vi "KundtsTube.vi"() -> ()   [LabVIEW 2014]
panel:
  out "XY Graph":cluster{"Y":dbl[], "Y":dbl[]}[](graph)=[{"Y"=[10.0, 15.0, 20.0, 25.0, 30.0, 35.0, 40.0, 45.0, 50.0, 55.0, 60.0, 65.0, 70.0, 75.0, 80.0, 85.0, 90.0, 95.0, 100.0, 105.0, 110.0, 115.0, 120.0, 125.0, 130.0, 135.0, 140.0, 145.0, 150.0, 155.0, 160.0, 165.0, 170.0, 175.0, 180.0, 185.0, 190.0, 195.0, 200.0, 205.0, 210.0, 215.0, 220.0, 225.0, 230.0, 235.0, 240.0, 245.0, 250.0, 255.0, 260.0, 265.0, 270.0, 275.0, 280.0, 285.0, 290.0, 295.0, 300.0, 305.0, 310.0, 315.0, 320.0, 325.0, 330.0, 335.0, 340.0, 345.0, 350.0, 355.0, 360.0, 365.0, 370.0, 375.0, 380.0, 385.0, 390.0, 395.0, 400.0, 405.0, 410.0, 415.0, 420.0, 425.0, 430.0, 435.0, 440.0, 445.0, 450.0, 455.0, 460.0, 465.0, 470.0, 475.0, 480.0, 485.0, 490.0, 495.0, 500.0, 505.0, 510.0, 515.0, 520.0], "Y"=[0.04456068816861268, 0.04246761801420257, 0.0029318464951392296, 0.006187733700200648, 0.025257929686987424, 0.006652860441749366, 0.01153669119734088, 0.00781567729339892, 0.01781590208649467, 0.01060643772440381, 0.08781746904711077, 0.23572771854025024, 0.016653085262158942, 0.01804846545098053, 0.02502536632644286, 0.060607559009512875, 0.04921195514147016, 0.024327676244046137, 0.026420746487802522, 0.031304577016499566, 0.03363021058187243, 0.035723280779826894, 0.04037454784947645, 0.04618863161490958, 0.05642141884865977, 0.07177059923637953, 0.07665442924315613, 0.10688766136403363, 0.12014377015038061, 0.1582841510008175, 0.22991363739015455, 0.3892194315388213, 0.6971329375854346, 0.537594699872119, 0.3243343052383702, 0.22875082115043496, 0.18130791581667072, 0.15107468903161841, 0.1292137390800751, 0.11712044713048636, 0.10758535131053182, 0.10200383170628566, 0.09479436877503437, 0.09130591892545796, 0.09084079227667378, 0.08758490572086486, 0.08618952576070507, 0.08758490572086486, 0.08665465241460296, 0.08851515902508146, 0.0892128490019016, 0.09363155216170617, 0.09688743867096686, 0.10270152166084855, 0.1080504779408904, 0.11642275719974288, 0.13339987852029553, 0.13619063812401394, 0.15572595483233767, 0.17293563784776525, 0.2013083569553088, 0.2410766731269191, 0.3003802954713808, 0.3920101894309352, 0.538292389094699, 0.709458775490021, 0.6908537369984933, 0.524106041334506, 0.3906148104872364, 0.3075897548669105, 0.2538676512086395, 0.21619240555553426, 0.18944763034861226, 0.17200538472980892, 0.15572595483233767, 0.14502804341384531, 0.1380511445162259, 0.1299114289896649, 0.12549272620943444, 0.12270196653491103, 0.12014377015038061, 0.1187483902977361, 0.12060889676690342, 0.12060889676690342, 0.12479503629253452, 0.12270196653491103, 0.1280509225615268, 0.13270218861647873, 0.15898184086224848, 0.1780520299597052, 0.1587492775752334, 0.1743310175208379, 0.19177326304302644, 0.21572727904478303, 0.2510768923878622, 0.30014773226299196, 0.37991690509556547, 0.4913146454467467, 0.6422480698909717, 0.7580644344885081, 0.6671323116767275, 0.522245536673662, 0.38526585782603767]}]
  out "Frequency":i32=520
  in  "Minimum":i32=10
  in  "Maximum":i32=10000
  in  "# of Points":i32=1999
  in  "Spacing":enum16{"Linear", "Logrithmic"}(ring)
  in  "Tab Control":enum32{"Sweep", "Single"}(tab)
  in  "Seconds to Wait":u32=1
  in  "Frequency":i32
  out "RMS":dbl=0.38526585782603767
  in  "# of Samples":dbl=10000.0
  in  "Sampling Rate":dbl=100000.0
  in  "Amplitude":i32=2
  in  "stop":bool
  out "Waveform Graph":dynamicdata(graph)=[{"t0"=timestamp(3497994291.28955 s since 1904-01-01), "dt"=9.999999999999972e-06, "Y"=array[10000 elements], "attributes"=variant("NI_ChannelName"=variant(string "Voltage"), "NI_UnitDescription"=variant(string "Volts"))}]
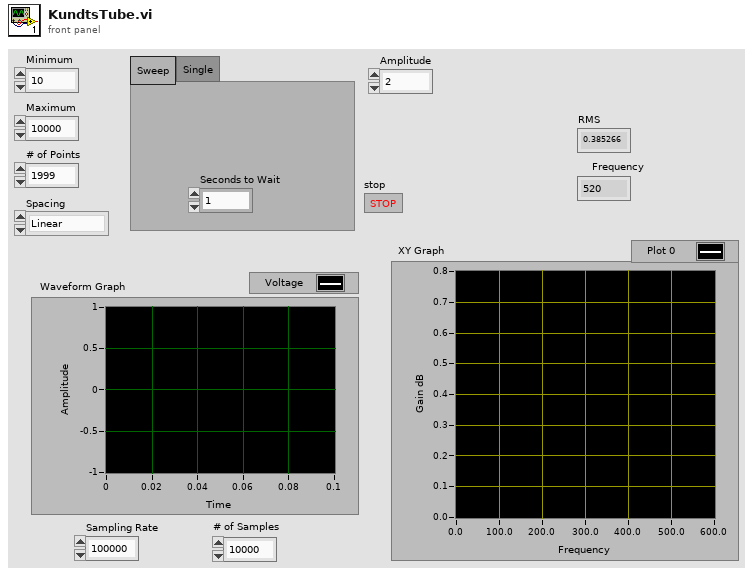
[diagram p1: front panel]
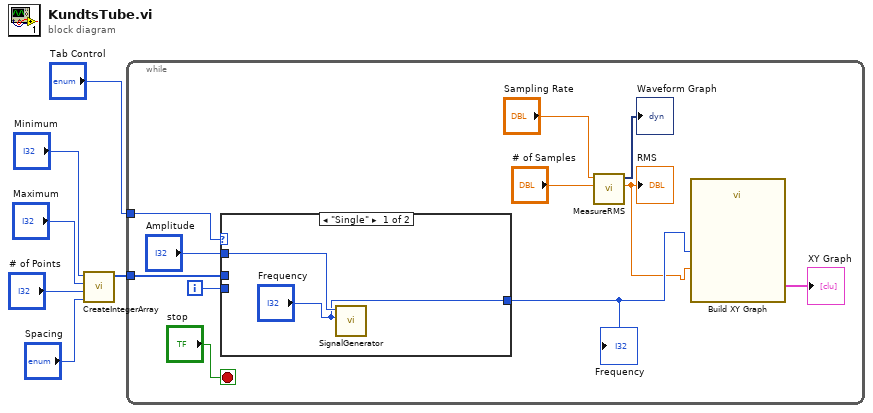
[diagram p0: block diagram]
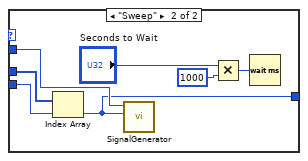
[diagram p2: hidden frame]
diagram:
  n1 = call "CreateIntegerArray.vi"("Spacing"="Spacing", "# of Points"="# of Points", "Maximum"="Maximum", "Minimum"="Minimum") -> ("Array"=w1:i32[])  [unwired: 7 in]
  n2 = while {
    tunnel: w1 -> [w11]
    tunnel: "Tab Control" -> [w14]
    i -> [w15]
    stop <- "stop" stop-if-true
    n3 = case shown="\"Single\"" w14 {
      tunnel: "Amplitude" -> [w19 w21]
      tunnel: w15 -> [_ w23]
      tunnel: w11 -> [_ w22]
      tunnel: ["Frequency" w20] -> w8
      frame "Single" {
        n4 = call "SignalGenerator.vi"("Frequency"="Frequency", "Amplitude"=w19) -> ()  [unwired: 9 in, 1 out]
      }
      frame "Sweep" {
        n5 = Index Array(array=w22, index=w23) -> (element=w20:i32)
        n6 = call "SignalGenerator.vi"("Frequency"=w20, "Amplitude"=w21) -> ()  [unwired: 9 in, 1 out]
        n7 = Multiply(x="Seconds to Wait", y=1000) -> (x*y=w26:u32)
        n8 = Wait (ms)(milliseconds to wait=w26) -> ()  [unwired: 1 out]
      }
    }
    "Frequency" <- w8
    n9 = call "MeasureRMS.vi"("Sampling Rate"="Sampling Rate", "# of Samples"="# of Samples") -> ("Waveform Graph"=→"Waveform Graph":dynamicdata, "RMS"=w7:dbl)  [unwired: 7 in]
    "RMS" <- w7
    n10 = call "Build XY Graph"("Y Input"=w7, "X Input"=w8) -> ("XY Graph"=→"XY Graph":cluster{"X":dbl[], "Y":dbl[]}[])  [unwired: 8 in, 1 out]
  }
